vi "Write String.vi"(6 "error in (no error)":errorcluster, 7 "Bus In":refnum<class "Bus.lvclass">, 8 "Channel Name":string, 9 "Data Value Engineering":dbl, 10 "Data Value Native":dbl, 11 "All Channels in":refnum<class "All Channels Out.lvclass">) -> (0 "error out":errorcluster, 3 "All Channels out":refnum<class "All Channels Out.lvclass">, 5 "Bus Out":refnum<class "Bus.lvclass">)   [LabVIEW 2018, in "All Channels Out.lvclass"]
doc: "All Channels.lvclass:Read String.vi\n\nThis is the Read String VI forthe All Channels class.\n\nInstrument Communication Module Version 1.0\nOctober, 2020 Original Code Consulting Davita Bird\n www.originalcode.com"
uses:
  All Channels Out.lvclass
  Bus/Bus.lvclass
  All Channels Out.lvclass/All Channels Out.ctl
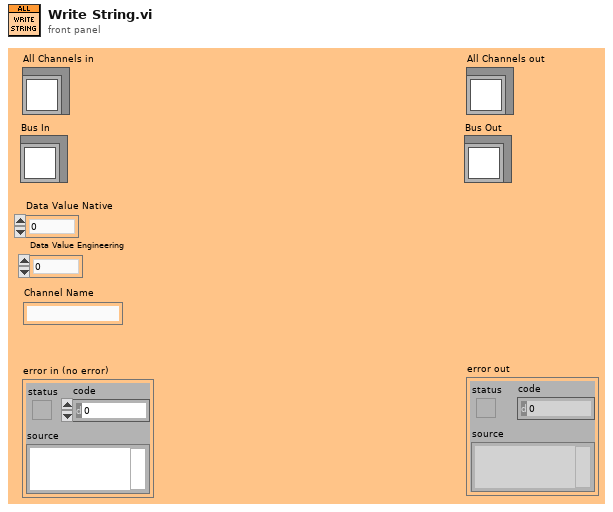
[diagram p1: front panel]
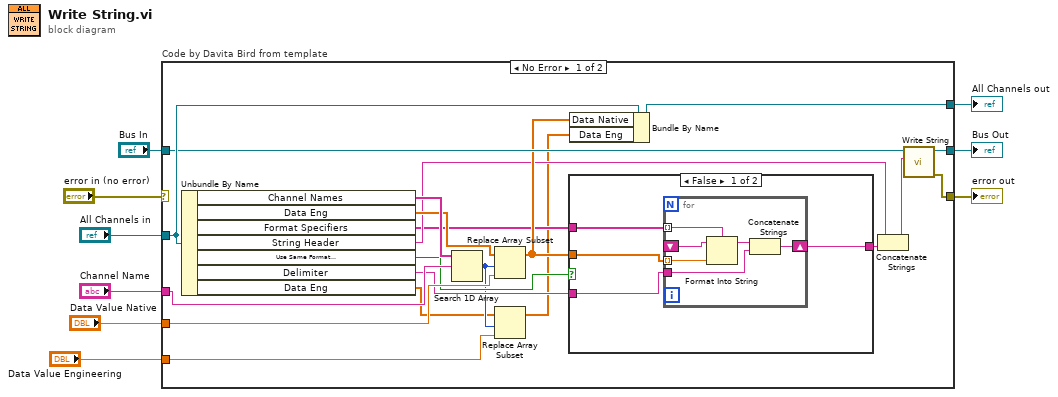
[diagram p0: block diagram]
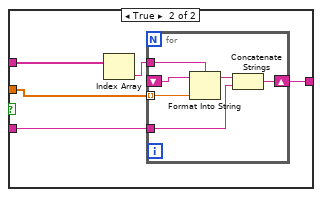
[diagram p2: hidden frame]
diagram:
  n1 = case "Code by Davita Bird from template" shown="No Error" "error in (no error)" {
    selector: "error in (no error)" -> [_ w53]
    tunnel: [w21 w53] -> w8
    tunnel: [w29 w52] -> w7
    tunnel: "All Channels in" -> [w28 w52]
    tunnel: "Data Value Native" -> [w24 _]
    tunnel: "Bus In" -> [w22 w51]
    tunnel: [w23 w51] -> w4
    tunnel: "Channel Name" -> [w26 _]
    tunnel: "Data Value Engineering" -> [w12 _]
    frame No Error {
      n2 = Unbundle By Name(w28) -> ("Channel Names"=w27:string[], "Data Eng"=w25:dbl[], "Format Specifiers"=w15:string[], "String Header"=w17:string, "Use Same Format\nSpecifier \nFor All Channels"=w20:bool, "Delimiter"=w16:string, "Data Eng"=w10:dbl[])
      n3 = Search 1D Array(1D array=w27, element=w26) -> (index of element=w11:i32)  [unwired: 1 in]
      n4 = Replace Array Subset(array=w25, new element=w24, index=w11) -> (w19:dbl[])
      n5 = Replace Array Subset(array=w10, new element=w12, index=w11) -> (w13:dbl[])
      n6 = case shown="False" w20 {
        tunnel: w19 -> [w32 w44]
        tunnel: [w30 w43] -> w18
        tunnel: w16 -> [w31 w42]
        tunnel: w15 -> [w33 w41]
        frame False {
          n7 = for {
            tunnel: w33 -> [w39] mode=indexing
            tunnel: w32 -> [w38] mode=indexing
            tunnel: w31 -> [w37]
            shift-right: [w35] -> w30
            shift-left: _ -> [w34]
            n8 = Format Into String(format string=w39, initial string=w34, w38) -> (resulting string=w36:string)  [unwired: 1 in, 1 out]
            n9 = Concatenate Strings(w36, w37) -> (w35:string)
          }
        }
        frame True {
          n10 = Index Array(array=w41) -> (element=w40:string)  [unwired: 1 in]
          n11 = for {
            tunnel: w44 -> [w49] mode=indexing
            tunnel: w40 -> [w50]
            shift-right: [w46] -> w43
            shift-left: _ -> [w47]
            tunnel: w42 -> [w45]
            n12 = Format Into String(format string=w50, initial string=w47, w49) -> (resulting string=w48:string)  [unwired: 1 in, 1 out]
            n13 = Concatenate Strings(w48, w45) -> (w46:string)
          }
        }
      }
      n14 = Bundle By Name(cluster=w28, "Data Native"=w19, "Data Eng"=w13) -> (w29:refnum<class "All Channels Out.lvclass">)
      n15 = Concatenate Strings(w17, w18) -> (w14:string)
      n16 = call-dynamic "Write String.vi"("String"=w14, "Bus in"=w22) -> ("error out"=w21:errorcluster, "Bus out"=w23:refnum<class "Bus.lvclass">)  [unwired: 8 in]
    }
    frame Error {
    }
  }
  "error out" <- w8
  "All Channels out" <- w7
  "Bus Out" <- w4
